vi "lee_todo_ajustes_previos.vi"(8 "error in (no error)":errorcluster, 11 "Base de Datos in":refnum<class "Base de Datos.lvclass">) -> (0 "error out":errorcluster, 3 "Base de Datos out":refnum<class "Base de Datos.lvclass">)   [LabVIEW 2019, in "Base de Datos.lvclass"]
uses:
  Base de Datos.lvclass
  SQLiteConnector/SQLiteConnection.lvclass
panel:
  in  "Tipo Equipo":enum16{"Sonometro", "Calibrador", "Dosimetro"}(ring)
  out "result":string[][](array[string])
  out "query":string
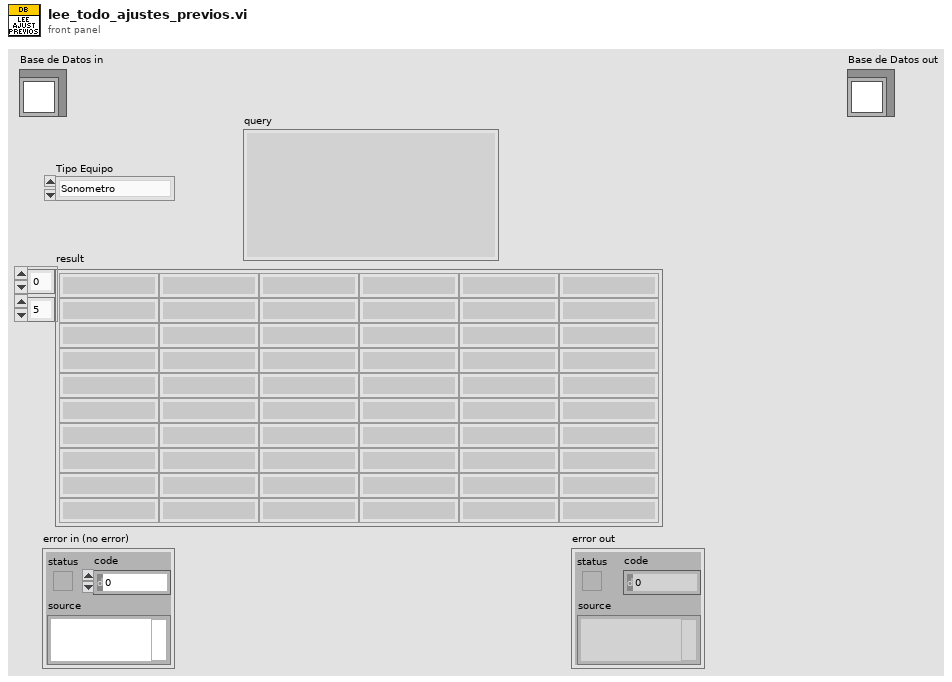
[diagram p1: front panel]
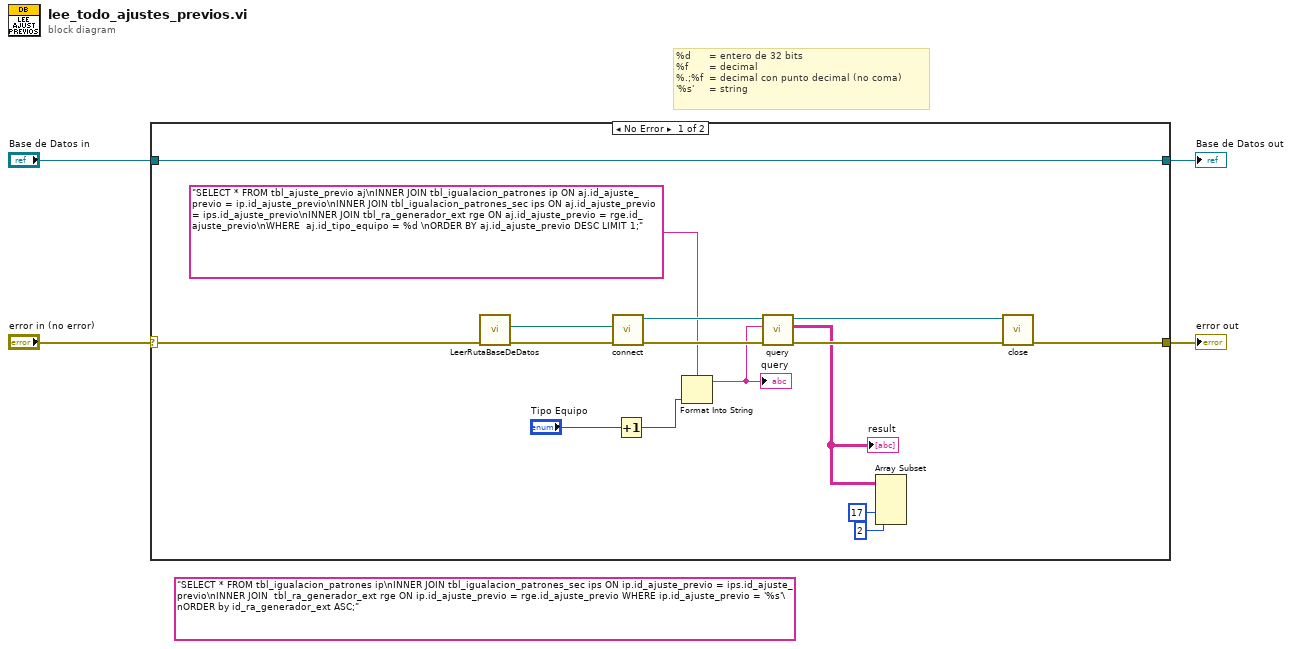
[diagram p0: block diagram]
diagram:
  (unwired) "SELECT * FROM tbl_igualacion_patrones ip\nINNER JOIN tbl_igualacion_patrones_sec ips ON ip.id_ajuste_previo = ips.id_ajuste_previo\nINNER JOIN  tbl_ra_generador_ext rge ON ip.id_ajuste_previo = rge.id_ajuste_previo WHERE ip.id_ajuste_previo = '%s'\nORDER by id_ra_generador_ext ASC;" ("format string")
  # "%d      = entero de 32 bits\n%f       = decimal\n%.;%f  = decimal con punto decimal (no coma)\n'%s'     = string"
  n1 = case shown="No Error" "error in (no error)" {
    selector: "error in (no error)" -> [w11 w21]
    tunnel: [w18 w21] -> w4
    tunnel: "Base de Datos in" -> [w12 w22]
    tunnel: [w12 w22] -> w1
    frame No Error {
      n2 = call "LeerRutaBaseDeDatos.vi"("error in (no error)"=w11) -> ("error out"=w10:errorcluster, "Database Path"=w9:path)  [unwired: 9 in]
      n3 = call "connect.vi"("error in (no error)"=w10, "Database Path"=w9) -> ("error out"=w20:errorcluster, "object out"=w13:refnum<class "SQLiteConnection.lvclass">)  [unwired: 8 in]
      n4 = Increment(x="Tipo Equipo") -> (x+1=w6:enum16{"Sonometro", "Calibrador", "Dosimetro"})
      n5 = Format Into String(format string="SELECT * FROM tbl_ajuste_previo aj\nINNER JOIN tbl_igualacion_patrones ip ON aj.id_ajuste_previo = ip.id_ajuste_previo\nINNER JOIN tbl_igualacion_patrones_sec ips ON aj.id_ajuste_previo = ips.id_ajuste_previo\nINNER JOIN tbl_ra_generador_ext rge ON aj.id_ajuste_previo = rge.id_ajuste_previo\nWHERE  aj.id_tipo_equipo = %d \nORDER BY aj.id_ajuste_previo DESC LIMIT 1;", w6) -> (resulting string=w5:string)  [unwired: 2 in, 1 out]
      "query" <- w5
      n6 = call "query.vi"("error in (no error)"=w20, "SQL Statement"=w5, "object in"=w13) -> ("error out"=w19:errorcluster, "result"=w16:string[][], "object out"=w17:refnum<class "SQLiteConnection.lvclass">)  [unwired: 5 in, 1 out]
      "result" <- w16
      n7 = Array Subset(array=w16, index (col)=17 ("index"), length (col)=2 ("length")) -> ()  [unwired: 2 in, 1 out]
      n8 = call-dynamic "close.vi"("error in (no error)"=w19, "object in"=w17) -> ("error out"=w18:errorcluster)  [unwired: 8 in, 1 out]
    }
    frame Error {
    }
  }
  "error out" <- w4
  "Base de Datos out" <- w1
